vi "Disconnect from Server.vi"(8 "error in (no error)":errorcluster, 11 "Client in":refnum<class "Client.lvclass">) -> (0 "error out":errorcluster, 1 "timed out":bool, 3 "Client out":refnum<class "Client.lvclass">)   [LabVIEW 2013, in "MQTT Client.lvlib" / "Client.lvclass"]
uses:
  Client.lvclass
  Client.lvclass/Client.ctl
  MQTT_Base/Session/Session.lvclass/Session.ctl
  <vilib>/LabVIEW Open Source Project/MQTT Control Packets/Control Packets/DISCONNECT/DISCONNECT.lvclass
  Session.Client/Session.Client.lvclass
  MQTT_Base/Session/Session.lvclass
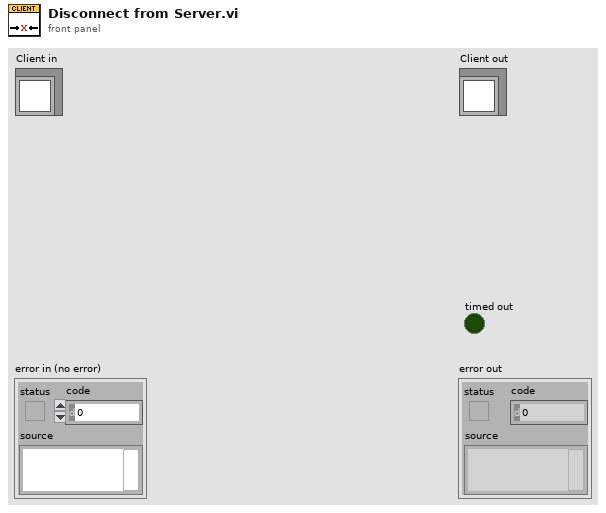
[diagram p1: front panel]
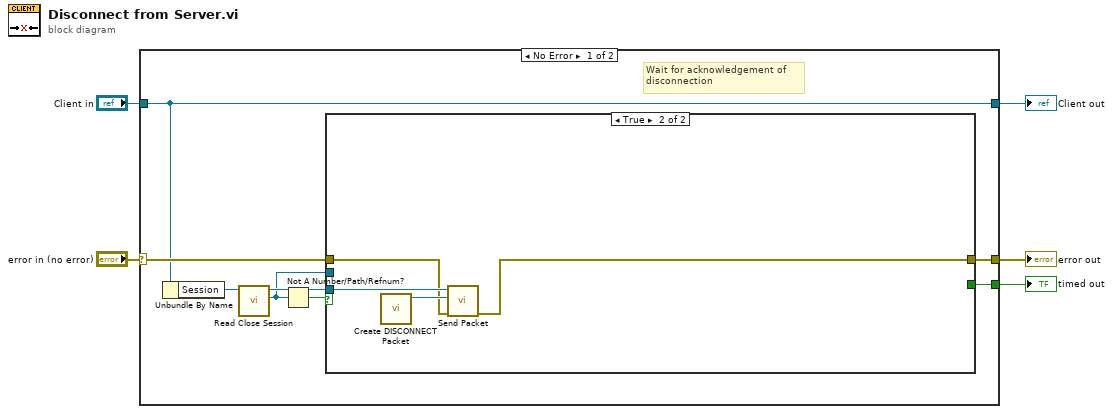
[diagram p0: block diagram]
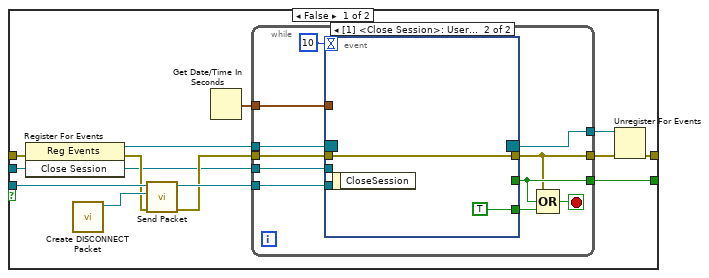
[diagram p2: hidden frame]
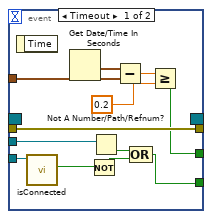
[diagram p3: hidden frame]
diagram:
  n1 = case shown="No Error" "error in (no error)" {
    selector: "error in (no error)" -> [w13 w57]
    tunnel: [w12 w57] -> w4
    tunnel: [w10 w56] -> w2
    tunnel: "Client in" -> [w10 w56]
    tunnel: [w11 _] -> w1
    frame No Error {
      # "Wait for acknowledgement of\ndisconnection"
      n2 = Unbundle By Name(w10) -> ("Session"=w8:refnum<class "Session.Client.lvclass">)
      n3 = call "Read Close Session.vi"("Session in"=w8) -> ("Close Session"=w6:refnum<user-event>, "Session out"=w7:refnum<class "Session.Client.lvclass">)  [unwired: 8 in, 1 out]
      n4 = Not A Number/Path/Refnum?(number/path/refnum=w6) -> (NaN/Path/Refnum?=w9:bool)
      n5 = case shown="True" w9 {
        tunnel: w13 -> [w26 w53]
        tunnel: [w25 w52] -> w12
        tunnel: [w24 _] -> w11
        tunnel: w7 -> [w18 w54]
        tunnel: w6 -> [w14 _]
        frame False {
          n6 = register-events(error in=w26, w14) -> (reference out=w21:refnum<event-registration>, error out=w16:errorcluster)  [unwired: 1 in]
          n7 = call <vilib>:"Create DISCONNECT Packet.vi"() -> ("DISCONNECT"=w19:refnum<class "DISCONNECT.lvclass">)  [unwired: 9 in, 2 out]
          n8 = call "Send Packet.vi"("error in (no error)"=w16, "Packet"=w19, "Session"=w18) -> ("error out"=w15:errorcluster, "Session"=w17:refnum<class "Session.Client.lvclass">)  [unwired: 5 in, 2 out]
          n9 = Get Date/Time In Seconds() -> (seconds since 1Jan1904=w20:timestamp)
          n10 = while {
            tunnel: [w31] -> w24
            tunnel: [w37] -> w23
            tunnel: [w30] -> w22
            tunnel: w15 -> [w36]
            tunnel: w21 -> [w35]
            tunnel: w17 -> [w29]
            tunnel: w14 -> [w28]
            tunnel: w20 -> [w27]
            stop <- w32 stop-if-true
            n11 = event shown="[1] <Close Session>: User Event" {
              selector: w35 -> [_ _]
              dyn-events: [_ _] -> w37
              timeout: 10 -> [_ _]
              tunnel: [w49 w51] -> w30
              tunnel: w36 -> [w49 w51]
              tunnel: [w46 _] -> w31
              tunnel: [w42 TRUE] -> w33
              tunnel: w29 -> [w41 _]
              tunnel: w28 -> [w45 _]
              tunnel: w27 -> [w38 _]
              event Timeout {
                n12 = event-data() -> ()  [unwired: 1 in, 1 out]
                n13 = call "isConnected.vi"("Session in"=w41) -> ("connected"=w40:bool)  [unwired: 8 in, 2 out]
                n14 = Get Date/Time In Seconds() -> (seconds since 1Jan1904=w39:timestamp)
                n15 = Not(x=w40) -> (.not. x?=w43:bool)
                n16 = Not A Number/Path/Refnum?(number/path/refnum=w45) -> (NaN/Path/Refnum?=w44:bool)
                n17 = Subtract(x=w39, y=w38) -> (x-y=w48:dbl)
                n18 = Compound Arithmetic op=OR(w44, w43) -> (w42:bool)
                n19 = Greater Or Equal?(x=w48, y=0.2) -> (x >= y?=w46:bool)
              }
              event User Event {
                n20 = event-data() -> ()  [unwired: 1 in, 1 out]
              }
            }
            n21 = Compound Arithmetic op=OR(w30, w31, w33) -> (w32:bool)
          }
          n22 = Unregister For Events(event registration refnum=w23, error in=w22) -> (error out=w25:errorcluster)
        }
        frame True {
          n23 = call <vilib>:"Create DISCONNECT Packet.vi"() -> ("DISCONNECT"=w55:refnum<class "DISCONNECT.lvclass">)  [unwired: 9 in, 2 out]
          n24 = call "Send Packet.vi"("error in (no error)"=w53, "Packet"=w55, "Session"=w54) -> ("error out"=w52:errorcluster)  [unwired: 5 in, 3 out]
        }
      }
    }
    frame Error {
    }
  }
  "error out" <- w4
  "Client out" <- w2
  "timed out" <- w1
